vi "Get Resistance Waveform.vi"(9 "Config":T1={"Voltage Index"=1, "Current Index"=2, "Channel name"="Source-Current"}, 11 "array":waveform(dbl)[](array[waveform])) -> (1 "Voltage channel name":string, 3 "waveform out":waveform(dbl))   [LabVIEW 2019]
doc: "This example demonstrates how to acquire a continuous amount of data (Waveform) using the DAQ device's internal clock. It also shows how to synchronize two devices for different device families (E Series, S Series, M Series, X Series, DSA, and SC Express), to simultaneously acquire the data.\n\nFor instructions on how to connect your signals to the DAQ device, refer to your device documentation."
panel:
  out "Current channel name":string
  # "Get Power Waveform"
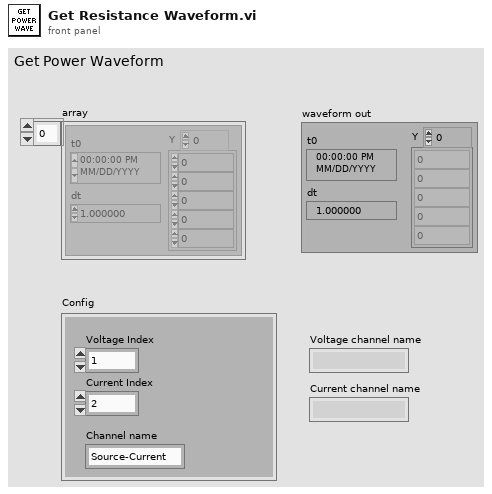
[diagram p1: front panel]
types:
  T1 = cluster{"Voltage Index":i32, "Current Index":i32, "Channel name":string}
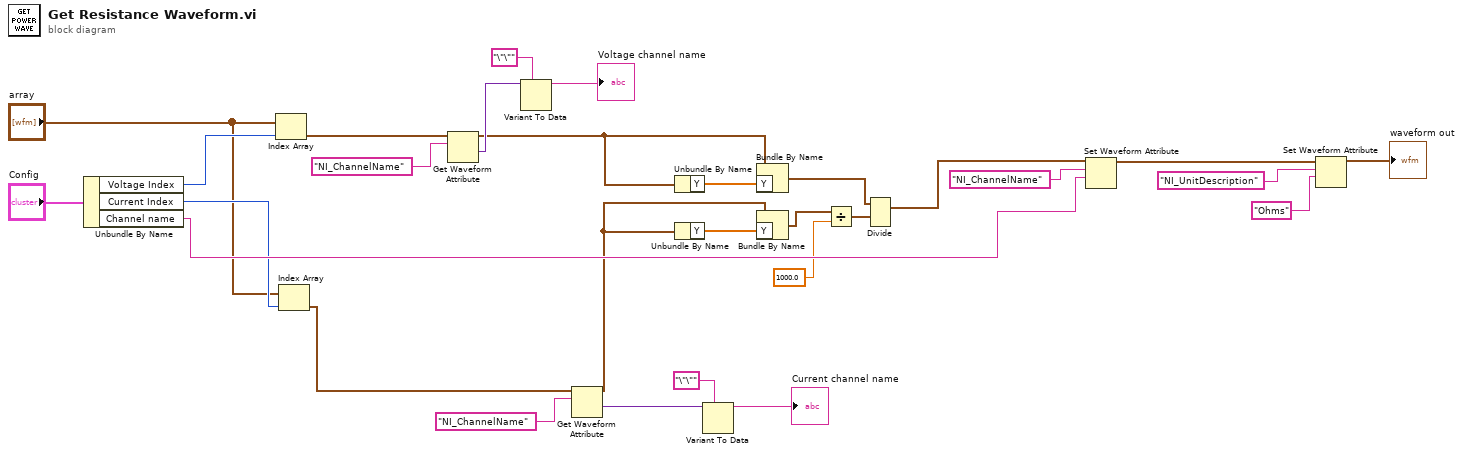
[diagram p0: block diagram]
diagram:
  n1 = Unbundle By Name("Config") -> ("Voltage Index"=w21:i32, "Current Index"=w13:i32, "Channel name"=w15:string)
  n2 = Index Array(array="array", index=w21) -> (element=w25:waveform(dbl))
  n3 = Index Array(array="array", index=w13) -> (element=w8:waveform(dbl))
  n4 = Get Waveform Attribute(6:"NI_ChannelName" ("name"), 7:w25) -> (1:w19:variant, 3:w17:waveform(dbl))  [unwired: 2 in, 2 out]
  n5 = Variant To Data(type="\"\"" ("name"), Variant=w19) -> (data=→"Voltage channel name":string)  [unwired: 1 in, 1 out]
  n6 = Get Waveform Attribute(6:"NI_ChannelName" ("name"), 7:w8) -> (1:w9:variant, 3:w4:waveform(dbl))  [unwired: 2 in, 2 out]
  n7 = Unbundle By Name(w17) -> ("Y"=w16:dbl[])
  n8 = Unbundle By Name(w4) -> ("Y"=w5:dbl[])
  n9 = Variant To Data(type="\"\"" ("name"), Variant=w9) -> (data=→"Current channel name":string)  [unwired: 1 in, 1 out]
  n10 = Bundle By Name(cluster=w17, "Y"=w16) -> (w6:waveform(dbl))
  n11 = Bundle By Name(cluster=w4, "Y"=w5) -> (w3:waveform(dbl))
  n12 = Divide(x=w3, y=1000.0) -> (x/y=w2:waveform(dbl))
  n13 = Divide(1:w2, 2:w6) -> (0:w14:waveform(dbl))  [unwired: 1 in, 1 out]
  n14 = Set Waveform Attribute(5:w15, 6:"NI_ChannelName" ("name"), 7:w14) -> (3:w27:waveform(dbl))  [unwired: 1 in, 2 out]
  n15 = Set Waveform Attribute(5:"Ohms" ("name"), 6:"NI_UnitDescription" ("name"), 7:w27) -> (3:→"waveform out":waveform(dbl))  [unwired: 1 in, 2 out]
